vi "SaveFrameToPNG.vi"(7 "Save Image?":bool, 8 "Block Folder":path, 9 "Subfolder":string="Eyetracker", 10 "Refnum in":T1) -> (2 "Refnum out (duplicate)":T1, 3 "ImageSaved":bool=TRUE)   [LabVIEW 2013]
uses:
  <vilib>/vision/Image Controls.llb/IMAQ Image.ctl
  <vilib>/vision/NI_Vision_Development_Module.lvlib
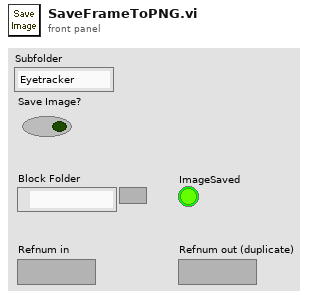
[diagram p1: front panel]
types:
  T1 = typedef "IMAQ Image.ctl" = refnum<image>
  T2 = cluster{"Desired Font (Application)":enum16{"User-specified Font", "Application Font", "System Font", "Dialog Font"}, "[User-specified Font]":cluster{"Font Name":string, "Size":i16, "Strikeout?":bool, "Italic?":bool, "Underline?":bool, "Outline?":bool, "Shadow?":bool, "Bold?":bool, "Rotation Angle":dbl}, "Horizontal Alignment":i16, "Vertical Alignment":i16}
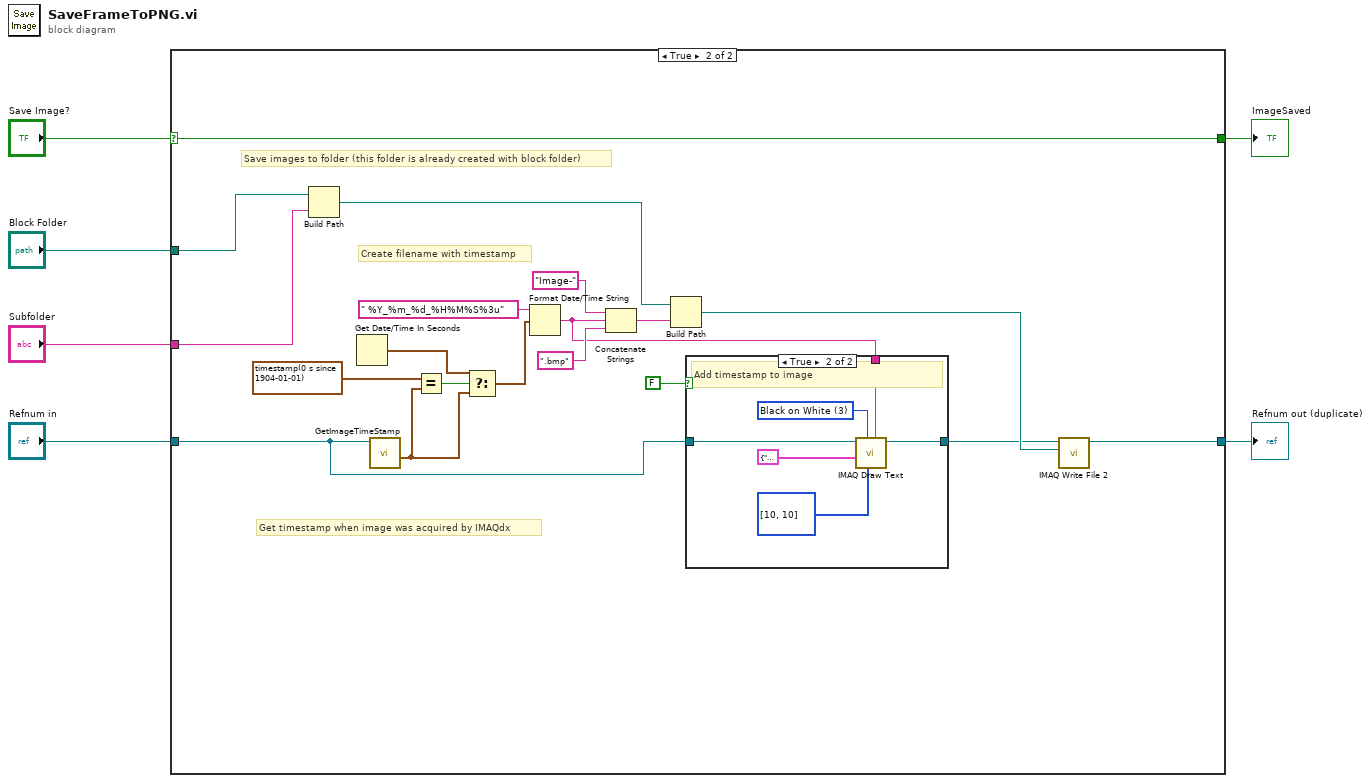
[diagram p0: block diagram]
diagram:
  n1 = case shown="True" "Save Image?" {
    selector: "Save Image?" -> [w7 w24]
    tunnel: [w8 w26] -> w6
    tunnel: "Block Folder" -> [_ w27]
    tunnel: "Refnum in" -> [w8 w25]
    tunnel: [w7 w24] -> w2
    tunnel: "Subfolder" -> [_ w23]
    frame False {
    }
    frame True {
      # "Get timestamp when image was acquired by IMAQdx"
      # "Save images to folder (this folder is already created with block folder)"
      # "Create filename with timestamp"
      n2 = Build Path(base path=w27, name or relative path=w23) -> (appended path=w17:path)
      n3 = Get Date/Time In Seconds() -> (seconds since 1Jan1904=w12:timestamp)
      n4 = call "GetImageTimeStamp.vi"("Image refnum in"=w25) -> ("System Time Stamp"=w11:timestamp)  [unwired: 9 in, 1 out]
      n5 = Equal?(x=timestamp(0 s since 1904-01-01), y=w11) -> (x = y?=w13:bool)
      n6 = Select(t=w12, s=w13, f=w11) -> (s? t:f=w10:timestamp)
      n7 = Format Date/Time String(time format string (%c)=" %Y_%m_%d_%H%M%S%3u", seconds (now)=w10) -> (date/time string=w16:string)  [unwired: 1 in]
      n8 = Concatenate Strings("Image-" ("string"), w16, ".bmp" ("string")) -> (w21:string)
      n9 = Build Path(base path=w17, name or relative path=w21) -> (appended path=w22:path)
      n10 = case shown="True" FALSE {
        tunnel: w16 -> [_ w34]
        tunnel: w25 -> [w28 w30]
        tunnel: [w28 w29] -> w14
        frame False {
        }
        frame True {
          w31 = 3 items=["White", "Black", "Inverted", "Black on White", "White on Black"] ("Color")
          # "Add timestamp to image"
          n11 = call "IMAQ Draw Text"("String"=w34, "Insertion Point"=i32[] [10, 10], "Color"=w31, "Font, Size & Style"=T2 {"Desired Font (Application)"=enum."User-specified Font", "[User-specified Font]"={"Font Name"="", "Size"=26, "Strikeout?"=FALSE, "Italic?"=FALSE, "Underline?"=FALSE, "Outline?"=FALSE, "Shadow?"=FALSE, "Bold?"=FALSE, "Rotation Angle"=0.0}, "Horizontal Alignment"=0, "Vertical Alignment"=1}, "Image Src"=w30) -> ("Image Dst Out"=w29:T1)  [unwired: 3 in, 3 out]
        }
      }
      n12 = call-poly "IMAQ Write File 2"("File Path"=w22, "Image"=w14) -> ("Image Out (duplicate)"=w26:T1)  [unwired: 8 in, 1 out]
    }
  }
  "Refnum out (duplicate)" <- w6
  "ImageSaved" <- w2
